vi "Clear CMD Reg.vi"(8 "error in (no error)":errorcluster, 11 "ModbusSp in":refnum<class "ModbusSp.lvclass">) -> (0 "error out":errorcluster, 3 "ModbusSp out":refnum<class "ModbusSp.lvclass">)   [LabVIEW 2019, in "ModbusSp.lvclass"]
uses:
  ModbusSp.lvclass
  ModbusSp.lvclass/ModbusSp.ctl
  <vilib>/NI/Modbus Library/API/Slave/Modbus Slave.lvclass
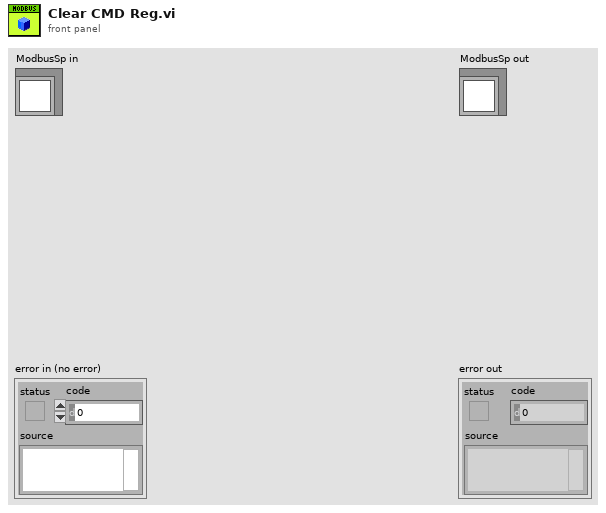
[diagram p1: front panel]
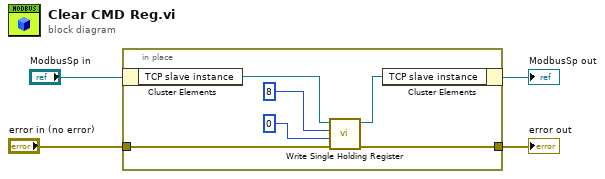
[diagram p0: block diagram]
diagram:
  n1 = in-place {
    in-place-border: "error in (no error)" -> [w8]
    in-place-border: [w7] -> w2
    n2 = in-place-cluster #1("ModbusSp in") -> ("TCP slave instance"=w10:refnum<class "Modbus Slave.lvclass">)
    n3 = call-dynamic "Write Single Holding Register.vi"("error in"=w8, "register to write"=u16 0, "address"=u16 8, "Modbus slave in"=w10) -> ("error out"=w7:errorcluster, "Modbus slave out"=w9:refnum<class "Modbus Slave.lvclass">)  [unwired: 6 in]
    n4 = in-place-cluster #1("TCP slave instance"=w9) -> (→"ModbusSp out":refnum<class "ModbusSp.lvclass">)
  }
  "error out" <- w2
